vi "GetSparkLine.vi"(0 "reference in":refnum<class "SparkLine.lvclass">, 5 "error in (no error)":errorcluster) -> (14 "reference out":refnum<class "SparkLine.lvclass">, 19 "error out":errorcluster)   [LabVIEW 2019, in "SparkLine.lvclass"]
doc: "Draws A button"
uses:
  SparkLine.lvclass
  C:/Users/Taylor.Hillegeist/OneDrive - Ultra/LabVIEW/Pgui2/Pgui_Obj_class/Pgui_Obj.lvclass
  Pgui_Obj_class/Pgui_Obj.lvclass
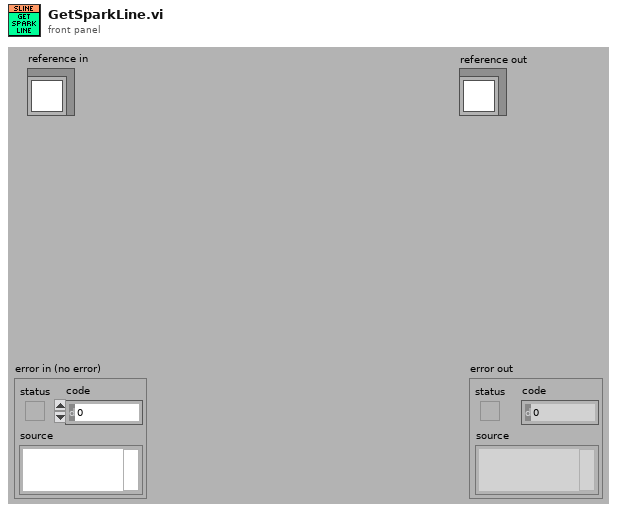
[diagram p1: front panel]
types:
  T1 = cluster{"left":i16, "top":i16, "right":i16, "bottom":i16}
  T2 = typedef "SparkLine.lvclass/ObjectAttributes.ctl" = cluster{"Override size":cluster{"Width":i16, "Height":i16}, "Data":dbl[]}
  T3 = typedef "Pgui_Obj.lvclass/ObjectAttributes.ctl" = cluster{"Children":refnum<class "Pgui_Obj.lvclass">[], "Draw Instr":picture, "Params":cluster{"left":i16, "top":i16, "right":i16, "bottom":i16}, "Parent_Pgui_Obj":refnum<class "Pgui_Obj.lvclass">, "MouseOver":bool}
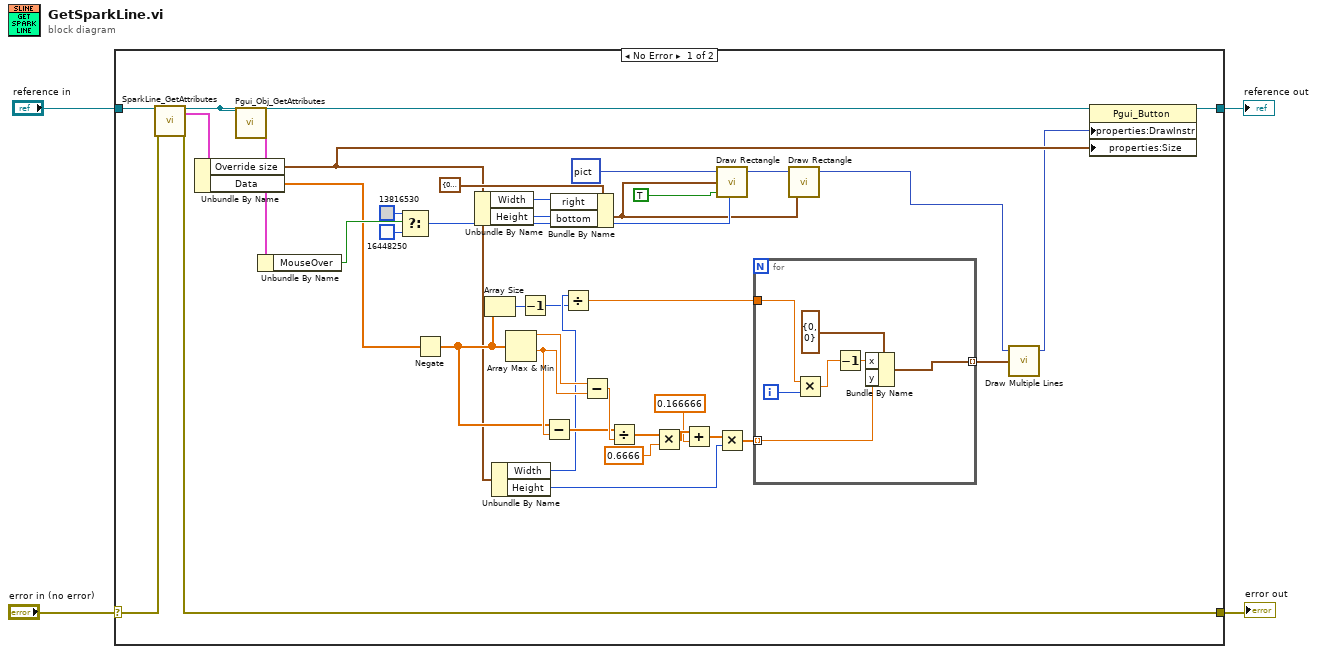
[diagram p0: block diagram]
diagram:
  n1 = case shown="No Error" "error in (no error)" {
    selector: "error in (no error)" -> [w43 w52]
    tunnel: [w41 w52] -> w3
    tunnel: [w37 w51] -> w1
    tunnel: "reference in" -> [w40 w51]
    frame No Error {
      n2 = call "SparkLine_GetAttributes.vi"("reference in"=w40, "error in (no error)"=w43) -> ("reference out"=w39:refnum<class "SparkLine.lvclass">, "Data"=w42:T2, "error out"=w41:errorcluster)  [unwired: 14 in, 1 out]
      n3 = Unbundle By Name(w42) -> ("Override size"=w8:cluster{"Width":i16, "Height":i16}, "Data"=w6:dbl[])
      n4 = call "Pgui_Obj_GetAttributes.vi"("reference in"=w39) -> ("Data"=w38:T3)  [unwired: 15 in, 3 out]
      n5 = Unbundle By Name(w38) -> ("MouseOver"=w9:bool)
      n6 = Select(t=u32 13816530 ("BG color(transparent)"), s=w9, f=u32 16448250 ("BG color(transparent)")) -> (s? t:f=w32:u32)
      n7 = Negate(x=w6) -> (-x=w10:dbl[])
      n8 = Unbundle By Name(w8) -> ("Width"=w26:i16, "Height"=w33:i16)
      n9 = Array Size(array=w10) -> (size(s)=w25:i32)
      n10 = Unbundle By Name(w8) -> ("Width"=w16:i16, "Height"=w19:i16)
      n11 = Array Max & Min(array=w10) -> (max value=w27:dbl, min value=w21:dbl)  [unwired: 2 out]
      n12 = Decrement(x=w25) -> (x-1=w5:i32)
      n13 = Subtract(x=w10, y=w21) -> (x-y=w20:dbl[])
      n14 = Bundle By Name(cluster=T1 {"left"=0, "top"=0, "right"=0, "bottom"=0} ("rect"), "right"=w26, "bottom"=w33) -> (w28:T1)
      n15 = Divide(x=w16, y=w5) -> (x/y=w17:dbl)
      n16 = Subtract(x=w27, y=w21) -> (x-y=w22:dbl)
      n17 = Divide(x=w20, y=w22) -> (x/y=w15:dbl[])
      n18 = Multiply(x=w15, y=0.6666) -> (x*y=w12:dbl[])
      n19 = Add(x=w12, y=0.166666) -> (x+y=w13:dbl[])
      n20 = call <vilib>:"Draw Rectangle.vi"("picture"=picture data[5B], "rect"=w28, "fill?(F)"=TRUE, "color(black)"=w32) -> ("new picture"=w29:picture)  [unwired: 5 in]
      n21 = Multiply(x=w13, y=w19) -> (x*y=w18:dbl[])
      n22 = for {
        tunnel: w17 -> [w46]
        tunnel: [w48] -> w24 mode=indexing
        tunnel: w18 -> [w47] mode=indexing
        i -> [w50]
        n23 = Multiply(x=w46, y=w50) -> (x*y=w45:dbl)
        n24 = Decrement(x=w45) -> (x-1=w44:dbl)
        n25 = Bundle By Name(cluster=cluster{"x":i16, "y":i16} {"x"=0, "y"=0}, "x"=w44, "y"=w47) -> (w48:cluster{"x":i16, "y":i16})
      }
      n26 = call <vilib>:"Draw Rectangle.vi"("picture"=w29, "rect"=w28) -> ("new picture"=w23:picture)  [unwired: 7 in]
      n27 = call <vilib>:"Draw Multiple Lines.vi"("picture"=w23, "line endpoints"=w24) -> ("new picture"=w7:picture)  [unwired: 7 in]
      n28 = property class="Pgui_Button"(reference=w39, "properties:DrawInstr"=w7, "properties:Size"=w8) -> (reference out=w37:refnum<class "SparkLine.lvclass">)  [unwired: 1 in, 1 out]
    }
    frame Error {
    }
  }
  "error out" <- w3
  "reference out" <- w1
